vi "Push.vi"(8 "Pair in":T1={"Давление заданное"=0.3, "Давление в системе"=99.99, "Расход заданый"=0.0, "Расход текущий"=0.0, "Объём заданный"=0.0, "Объём текущий"=0.0, "Старт давление"=FALSE, "Старт расход"=FALSE, "Сброс объёма"=FALSE, "plc_control"=FALSE, "lag_control"=FALSE, "mstop_control"=FALSE, "Давление"={"АЦП CH 0"=0.0, "АЦП CH 1"=0.0, "АЦП CH 2"=0.0, "АЦП CH 3"=0.0, "АЦП CH 4"=0.0, "АЦП CH 5"=0.0, "АЦП CH 6"=0.0, "АЦП CH 7"=0.0}, "Modbus"={"Массив чтения"=[], "Массив записи"=[]}} {"Давление"."АЦП CH 7" format="%.3f"; "Давление"."АЦП CH 6" format="%.3f"; "Давление"."АЦП CH 5" format="%.3f"; "Давление"."АЦП CH 4" format="%.3f"; "Давление"."АЦП CH 3" format="%.3f"; "Давление"."АЦП CH 2" format="%.3f"; "Давление"."АЦП CH 1" format="%.3f"; "Давление"."АЦП CH 0" format="%.3f"; "Объём текущий" min=0.0 max=9999.0 step=0.0001 format="%#_5f"; "Объём заданный" min=0.0 max=9999.0 step=0.0001 format="%#_5f"; "Расход текущий" format="%#_5f"; "Расход заданый" min=0.0 max=40.0 step=0.0001 format="%#_5f"; "Давление в системе" format="%.3f"; "Давление заданное" min=0.3 max=100.0 step=0.01 format="%#_5f"}, 9 "Port 2 in":T2={"Давление заданное"=0.3, "Давление MAX заданное"=100.0, "Давление в насосе"=0.0, "Давление в системе"=99.99, "Расход заданый"=0.0, "Расход текущий"=0.0, "Объём заданный"=0.0, "Объём текущий"=0.0, "Позиция насоса %"=0.0, "Ток двигателя"=0.0, "controlMsg"="", "Клапан k_sys"=FALSE, "Клапан k_res"=FALSE, "Клапан k_air"=FALSE, "Вверх"=FALSE, "Домой"=FALSE, "Вниз"=FALSE, "Старт расход"=FALSE, "Старт давление"=FALSE, "Сброс объёма"=FALSE, "Сброс давления Рсис"=FALSE, "Сброс давления Рнас"=FALSE, "Bits"={"plc_control"=FALSE, "lag_control"=FALSE, "mstop_control"=FALSE, "st_home"=FALSE, "error"=FALSE, "mstart"=FALSE, "pair"=FALSE, "startQ"=FALSE, "startP"=FALSE, "volume_Stop"=FALSE}} {"Ток двигателя" format="%#_5f"; "Расход текущий" format="%#_5f"; "Давление в системе" format="%.3f"; "Объём текущий" min=0.0 max=9999.0 step=0.0001 format="%#_5f"; "Объём заданный" min=0.0 max=9999.0 step=0.0001 format="%#_5f"; "Давление MAX заданное" min=0.0 max=100.0 step=0.01 format="%#_5f"; "Давление заданное" min=0.3 max=100.0 step=0.01 format="%#_5f"; "Расход заданый" min=0.0 max=40.0 step=0.0001 format="%#_5f"; "Давление в насосе" format="%.3f"; "Позиция насоса %" scale=0.0..100.0 scale format="%.2f"}, 10 "Port 1 in":T2={"Давление заданное"=0.3, "Давление MAX заданное"=100.0, "Давление в насосе"=0.0, "Давление в системе"=99.99, "Расход заданый"=0.0, "Расход текущий"=0.0, "Объём заданный"=0.0, "Объём текущий"=0.0, "Позиция насоса %"=0.0, "Ток двигателя"=0.0, "controlMsg"="", "Клапан k_sys"=FALSE, "Клапан k_res"=FALSE, "Клапан k_air"=FALSE, "Вверх"=FALSE, "Домой"=FALSE, "Вниз"=FALSE, "Старт расход"=FALSE, "Старт давление"=FALSE, "Сброс объёма"=FALSE, "Сброс давления Рсис"=FALSE, "Сброс давления Рнас"=FALSE, "Bits"={"plc_control"=FALSE, "lag_control"=FALSE, "mstop_control"=FALSE, "st_home"=FALSE, "error"=FALSE, "mstart"=FALSE, "pair"=FALSE, "startQ"=FALSE, "startP"=FALSE, "volume_Stop"=FALSE}} {"Ток двигателя" format="%#_5f"; "Расход текущий" format="%#_5f"; "Давление в системе" format="%.3f"; "Объём текущий" min=0.0 max=9999.0 step=0.0001 format="%#_5f"; "Объём заданный" min=0.0 max=9999.0 step=0.0001 format="%#_5f"; "Давление MAX заданное" min=0.0 max=100.0 step=0.01 format="%#_5f"; "Давление заданное" min=0.3 max=100.0 step=0.01 format="%#_5f"; "Расход заданый" min=0.0 max=40.0 step=0.0001 format="%#_5f"; "Давление в насосе" format="%.3f"; "Позиция насоса %" scale=0.0..100.0 scale format="%.2f"}, 11 "Управление ПЛК":T3) -> (0 "error out":errorcluster, 1 "Pair out":T1={"Давление заданное"=0.3, "Давление в системе"=99.99, "Расход заданый"=0.0, "Расход текущий"=0.0, "Объём заданный"=0.0, "Объём текущий"=0.0, "Старт давление"=FALSE, "Старт расход"=FALSE, "Сброс объёма"=FALSE, "plc_control"=FALSE, "lag_control"=FALSE, "mstop_control"=FALSE, "Давление"={"АЦП CH 0"=0.0, "АЦП CH 1"=0.0, "АЦП CH 2"=0.0, "АЦП CH 3"=0.0, "АЦП CH 4"=0.0, "АЦП CH 5"=0.0, "АЦП CH 6"=0.0, "АЦП CH 7"=0.0}, "Modbus"={"Массив чтения"=[], "Массив записи"=[]}} {"Давление"."АЦП CH 7" format="%.3f"; "Давление"."АЦП CH 6" format="%.3f"; "Давление"."АЦП CH 5" format="%.3f"; "Давление"."АЦП CH 4" format="%.3f"; "Давление"."АЦП CH 3" format="%.3f"; "Давление"."АЦП CH 2" format="%.3f"; "Давление"."АЦП CH 1" format="%.3f"; "Давление"."АЦП CH 0" format="%.3f"; "Объём текущий" min=0.0 max=9999.0 step=0.0001 format="%#_5f"; "Объём заданный" min=0.0 max=9999.0 step=0.0001 format="%#_5f"; "Расход текущий" format="%#_5f"; "Расход заданый" min=0.0 max=40.0 step=0.0001 format="%#_5f"; "Давление в системе" format="%.3f"; "Давление заданное" min=0.3 max=100.0 step=0.01 format="%#_5f"}, 2 "Port 2 out":T2={"Давление заданное"=0.3, "Давление MAX заданное"=100.0, "Давление в насосе"=0.0, "Давление в системе"=99.99, "Расход заданый"=0.0, "Расход текущий"=0.0, "Объём заданный"=0.0, "Объём текущий"=0.0, "Позиция насоса %"=0.0, "Ток двигателя"=0.0, "controlMsg"="", "Клапан k_sys"=FALSE, "Клапан k_res"=FALSE, "Клапан k_air"=FALSE, "Вверх"=FALSE, "Домой"=FALSE, "Вниз"=FALSE, "Старт расход"=FALSE, "Старт давление"=FALSE, "Сброс объёма"=FALSE, "Сброс давления Рсис"=FALSE, "Сброс давления Рнас"=FALSE, "Bits"={"plc_control"=FALSE, "lag_control"=FALSE, "mstop_control"=FALSE, "st_home"=FALSE, "error"=FALSE, "mstart"=FALSE, "pair"=FALSE, "startQ"=FALSE, "startP"=FALSE, "volume_Stop"=FALSE}} {"Ток двигателя" format="%#_5f"; "Расход текущий" format="%#_5f"; "Давление в системе" format="%.3f"; "Объём текущий" min=0.0 max=9999.0 step=0.0001 format="%#_5f"; "Объём заданный" min=0.0 max=9999.0 step=0.0001 format="%#_5f"; "Давление MAX заданное" min=0.0 max=100.0 step=0.01 format="%#_5f"; "Давление заданное" min=0.3 max=100.0 step=0.01 format="%#_5f"; "Расход заданый" min=0.0 max=40.0 step=0.0001 format="%#_5f"; "Давление в насосе" format="%.3f"; "Позиция насоса %" scale=0.0..100.0 scale format="%.2f"}, 3 "Port 1 out":T2={"Давление заданное"=0.3, "Давление MAX заданное"=100.0, "Давление в насосе"=0.0, "Давление в системе"=99.99, "Расход заданый"=0.0, "Расход текущий"=0.0, "Объём заданный"=0.0, "Объём текущий"=0.0, "Позиция насоса %"=0.0, "Ток двигателя"=0.0, "controlMsg"="", "Клапан k_sys"=FALSE, "Клапан k_res"=FALSE, "Клапан k_air"=FALSE, "Вверх"=FALSE, "Домой"=FALSE, "Вниз"=FALSE, "Старт расход"=FALSE, "Старт давление"=FALSE, "Сброс объёма"=FALSE, "Сброс давления Рсис"=FALSE, "Сброс давления Рнас"=FALSE, "Bits"={"plc_control"=FALSE, "lag_control"=FALSE, "mstop_control"=FALSE, "st_home"=FALSE, "error"=FALSE, "mstart"=FALSE, "pair"=FALSE, "startQ"=FALSE, "startP"=FALSE, "volume_Stop"=FALSE}} {"Ток двигателя" format="%#_5f"; "Расход текущий" format="%#_5f"; "Давление в системе" format="%.3f"; "Объём текущий" min=0.0 max=9999.0 step=0.0001 format="%#_5f"; "Объём заданный" min=0.0 max=9999.0 step=0.0001 format="%#_5f"; "Давление MAX заданное" min=0.0 max=100.0 step=0.01 format="%#_5f"; "Давление заданное" min=0.3 max=100.0 step=0.01 format="%#_5f"; "Расход заданый" min=0.0 max=40.0 step=0.0001 format="%#_5f"; "Давление в насосе" format="%.3f"; "Позиция насоса %" scale=0.0..100.0 scale format="%.2f"})   [LabVIEW 2023, in "pump_Lib.lvlib"]
uses:
  pump_Lib.lvlib
  TypeDef/control_Type.ctl
  TypeDef/pump_Type.ctl
  TypeDef/pair_Type.ctl
  TypeDef/parametrs_Type.ctl
panel:
  # "%"
  # "%"
  # "%"
  # "%"
  # "%"
  # "%"
  # "%"
  # "%"
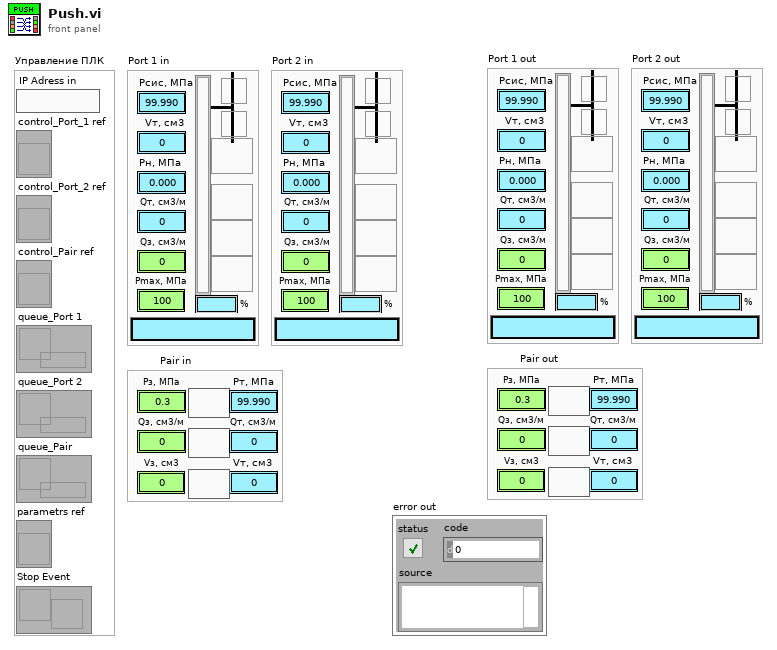
[diagram p1: front panel]
types:
  T1 = typedef "pump_Lib.lvlib/pair_Type.ctl" = cluster{"Давление заданное":dbl, "Давление в системе":dbl, "Расход заданый":dbl, "Расход текущий":dbl, "Объём заданный":dbl, "Объём текущий":dbl, "Старт давление":bool, "Старт расход":bool, "Сброс объёма":bool, "plc_control":bool, "lag_control":bool, "mstop_control":bool, "Давление":cluster{"АЦП CH 0":dbl, "АЦП CH 1":dbl, "АЦП CH 2":dbl, "АЦП CH 3":dbl, "АЦП CH 4":dbl, "АЦП CH 5":dbl, "АЦП CH 6":dbl, "АЦП CH 7":dbl}, "Modbus":cluster{"Массив чтения":u16[], "Массив записи":u16[]}}
  T2 = typedef "pump_Lib.lvlib/pump_Type.ctl" = cluster{"Давление заданное":dbl, "Давление MAX заданное":dbl, "Давление в насосе":dbl, "Давление в системе":dbl, "Расход заданый":dbl, "Расход текущий":dbl, "Объём заданный":dbl, "Объём текущий":dbl, "Позиция насоса %":dbl, "Ток двигателя":dbl, "controlMsg":string, "Клапан k_sys":bool, "Клапан k_res":bool, "Клапан k_air":bool, "Вверх":bool, "Домой":bool, "Вниз":bool, "Старт расход":bool, "Старт давление":bool, "Сброс объёма":bool, "Сброс давления Рсис":bool, "Сброс давления Рнас":bool, "Bits":cluster{"plc_control":bool, "lag_control":bool, "mstop_control":bool, "st_home":bool, "error":bool, "mstart":bool, "pair":bool, "startQ":bool, "startP":bool, "volume_Stop":bool}}
  T3 = typedef "pump_Lib.lvlib/control_Type.ctl" = cluster{"IP Adress in":string, "control_Port_1 ref":refnum<vi>, "control_Port_2 ref":refnum<vi>, "control_Pair ref":refnum<vi>, "queue_Port 1":refnum<queue>, "queue_Port 2":refnum<queue>, "queue_Pair":refnum<queue>, "parametrs ref":refnum<vi>, "Stop Event":refnum<user-event>}
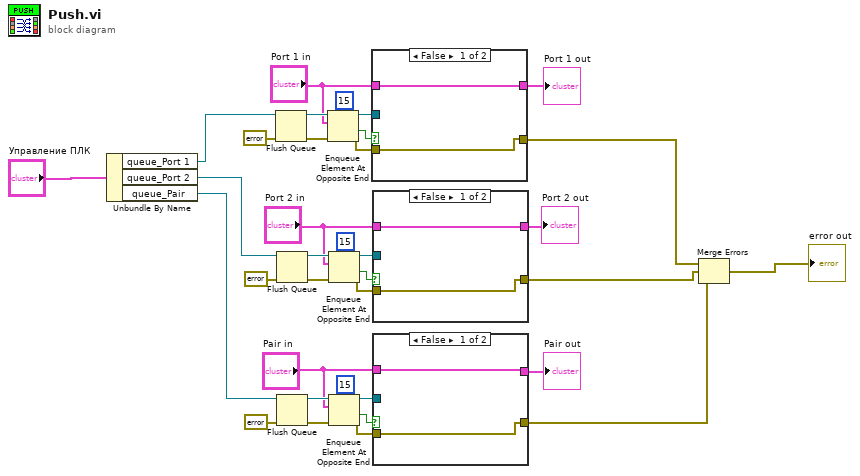
[diagram p0: block diagram]
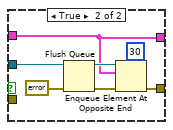
[diagram p2: hidden frame]
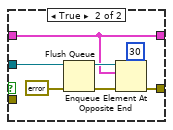
[diagram p3: hidden frame]
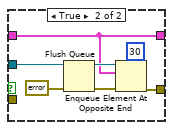
[diagram p4: hidden frame]
diagram:
  n1 = Unbundle By Name("Управление ПЛК") -> ("queue_Port 1"=w29:refnum<queue>, "queue_Port 2"=w14:refnum<queue>, "queue_Pair"=w11:refnum<queue>)
  n2 = Flush Queue(queue=w29, error in (no error)=errorcluster {"status"=FALSE, "code"=0, "source"=""}) -> (queue out=w35:refnum<queue>, error out=w34:errorcluster)  [unwired: 1 out]
  n3 = Flush Queue(queue=w14, error in (no error)=errorcluster {"status"=FALSE, "code"=0, "source"=""}) -> (queue out=w27:refnum<queue>, error out=w26:errorcluster)  [unwired: 1 out]
  n4 = Flush Queue(queue=w11, error in (no error)=errorcluster {"status"=FALSE, "code"=0, "source"=""}) -> (queue out=w22:refnum<queue>, error out=w21:errorcluster)  [unwired: 1 out]
  n5 = Enqueue Element At Opposite End(queue=w35, element="Port 1 in", timeout in ms (-1)=15, error in (no error)=w34) -> (queue out=w32:refnum<queue>, timed out?=w8:bool, error out=w7:errorcluster)
  n6 = Enqueue Element At Opposite End(queue=w27, element="Port 2 in", timeout in ms (-1)=15, error in (no error)=w26) -> (queue out=w24:refnum<queue>, timed out?=w9:bool, error out=w6:errorcluster)
  n7 = Enqueue Element At Opposite End(queue=w22, element="Pair in", timeout in ms (-1)=15, error in (no error)=w21) -> (queue out=w19:refnum<queue>, timed out?=w10:bool, error out=w5:errorcluster)
  n8 = case shown="False" w8 {
    tunnel: w32 -> [_ w43]
    tunnel: "Port 1 in" -> [w37 w39]
    tunnel: [w37 w39] -> w17
    tunnel: [w36 w38] -> w4
    tunnel: w7 -> [w36 _]
    frame False {
    }
    frame True {
      n9 = Flush Queue(queue=w43, error in (no error)=errorcluster {"status"=FALSE, "code"=0, "source"=""}) -> (queue out=w40:refnum<queue>, error out=w44:errorcluster)  [unwired: 1 out]
      n10 = Enqueue Element At Opposite End(queue=w40, element=w39, timeout in ms (-1)=30, error in (no error)=w44) -> (error out=w38:errorcluster)  [unwired: 2 out]
    }
  }
  "Port 1 out" <- w17
  n11 = case shown="False" w9 {
    tunnel: w24 -> [_ w52]
    tunnel: "Port 2 in" -> [w46 w48]
    tunnel: [w46 w48] -> w16
    tunnel: [w45 w47] -> w2
    tunnel: w6 -> [w45 _]
    frame False {
    }
    frame True {
      n12 = Flush Queue(queue=w52, error in (no error)=errorcluster {"status"=FALSE, "code"=0, "source"=""}) -> (queue out=w49:refnum<queue>, error out=w53:errorcluster)  [unwired: 1 out]
      n13 = Enqueue Element At Opposite End(queue=w49, element=w48, timeout in ms (-1)=30, error in (no error)=w53) -> (error out=w47:errorcluster)  [unwired: 2 out]
    }
  }
  "Port 2 out" <- w16
  n14 = case shown="False" w10 {
    tunnel: w19 -> [_ w61]
    tunnel: "Pair in" -> [w55 w57]
    tunnel: [w55 w57] -> w15
    tunnel: [w54 w56] -> w1
    tunnel: w5 -> [w54 _]
    frame False {
    }
    frame True {
      n15 = Flush Queue(queue=w61, error in (no error)=errorcluster {"status"=FALSE, "code"=0, "source"=""}) -> (queue out=w58:refnum<queue>, error out=w62:errorcluster)  [unwired: 1 out]
      n16 = Enqueue Element At Opposite End(queue=w58, element=w57, timeout in ms (-1)=30, error in (no error)=w62) -> (error out=w56:errorcluster)  [unwired: 2 out]
    }
  }
  "Pair out" <- w15
  n17 = Merge Errors(w4, w2, w1) -> (→"error out":errorcluster)
